vi "Limelight Vertical Position Control.vi"() -> ()   [LabVIEW 2020]
uses:
  <vilib>/Analysis/NI_AALPro.lvlib
panel:
  in  "V Correction \nFrom LimeLight":dbl
  in  "Target Distance\nFrom LimeLight":dbl
  in  "Kp":dbl
  in  "AutoTarget":bool
  in  "LimeLight Comm\nFailed":bool
  in  "LimeLight Target\nFound":bool
  out "Shooter Height\nAdjustment\nMotor":dbl
  out "Control\nStopped":bool
  out "Pv Adjustment\nFactor":dbl format="%0.2f"
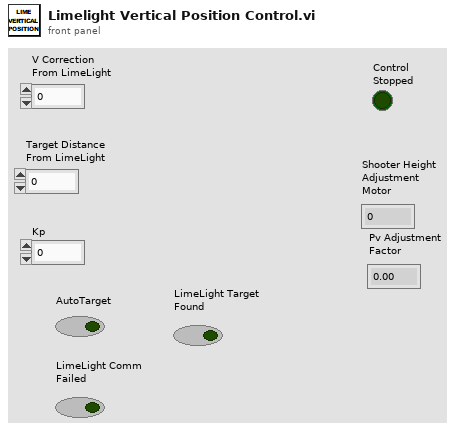
[diagram p1: front panel]
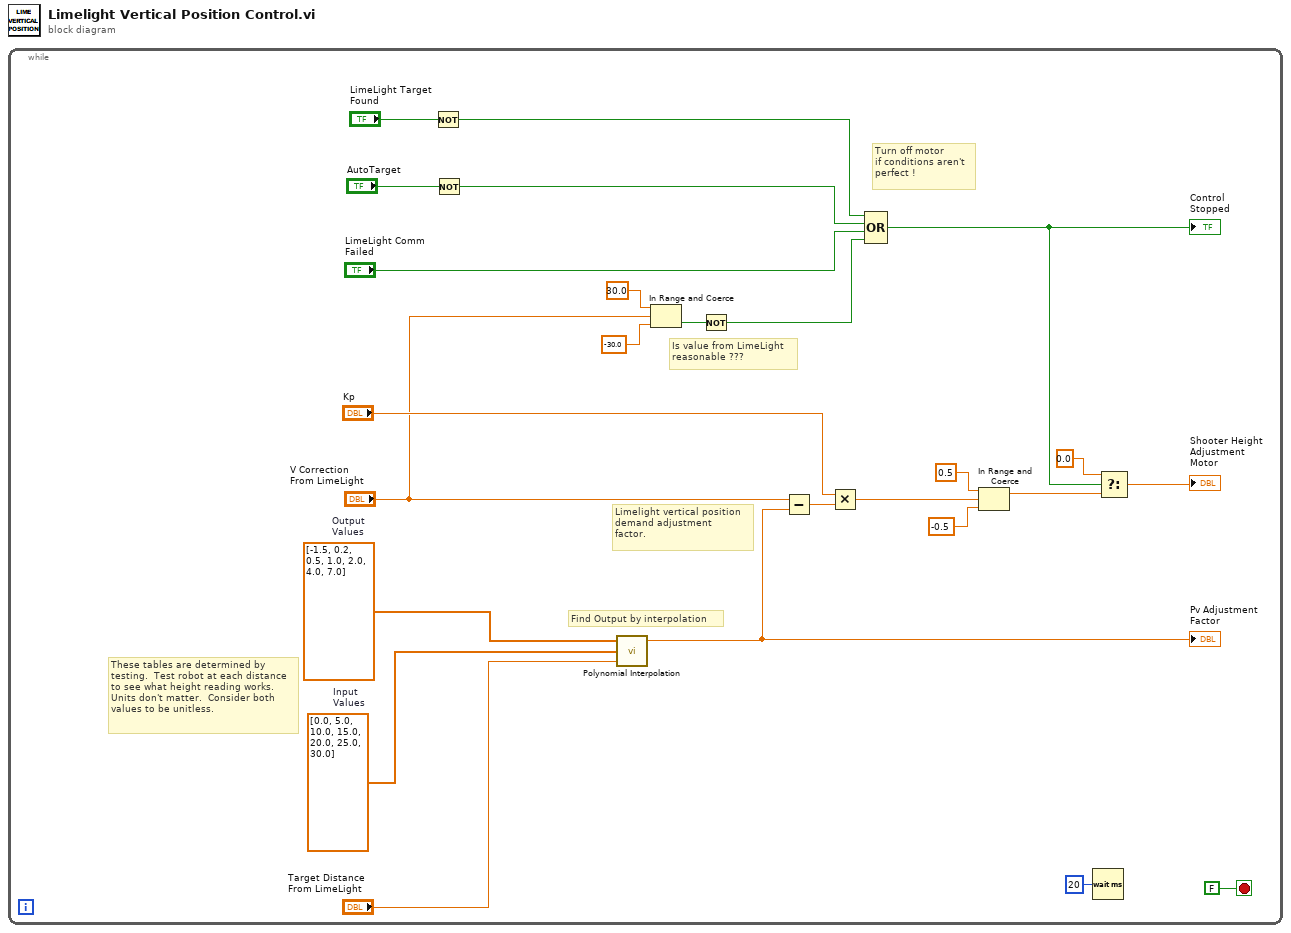
[diagram p0: block diagram]
diagram:
  n1 = while {
    stop <- FALSE stop-if-true
    w24 = dbl[] [0.0, 5.0, 10.0, 15.0, 20.0, 25.0, 30.0]  # Input  Values
    w25 = dbl[] [-1.5, 0.2, 0.5, 1.0, 2.0, 4.0, 7.0]  # Output  Values
    # "Turn off motor\nif conditions aren't\nperfect !"
    # "Is value from LimeLight\nreasonable ???"
    # "Limelight vertical position\ndemand adjustment \nfactor."
    # "These tables are determined by\ntesting.  Test robot at each distance\nto see what height reading works.\nUnits don't matter.  Consider both\nvalues to be unitless."
    # "Find Output by interpolation"
    n2 = Not(x="LimeLight Target\nFound") -> (.not. x?=w5:bool)
    n3 = Not(x="AutoTarget") -> (.not. x?=w14:bool)
    n4 = call <vilib>:"Polynomial Interpolation.vi"("x value"="Target Distance\nFrom LimeLight", "X"=w24, "Y"=w25) -> ("interpolation value"=w23:dbl)  [unwired: 2 out]
    "Pv Adjustment\nFactor" <- w23
    n5 = In Range and Coerce(upper limit=30.0, x="V Correction \nFrom LimeLight", lower limit=-30.0) -> (In Range?=w9:bool)  [unwired: 1 out]
    n6 = Not(x=w9) -> (.not. x?=w8:bool)
    n7 = Subtract(x="V Correction \nFrom LimeLight", y=w23) -> (x-y=w22:dbl)
    n8 = Multiply(x="Kp", y=w22) -> (x*y=w20:dbl)
    n9 = Compound Arithmetic op=OR(w5, w14, "LimeLight Comm\nFailed", w8) -> (w4:bool)
    "Control\nStopped" <- w4
    n10 = In Range and Coerce(upper limit=0.5, x=w20, lower limit=-0.5) -> (coerced(x)=w17:dbl)  [unwired: 1 out]
    n11 = Wait (ms)(milliseconds to wait=u32 20) -> ()  [unwired: 1 out]
    n12 = Select(t=0.0, s=w4, f=w17) -> (s? t:f=→"Shooter Height\nAdjustment\nMotor":dbl)
  }
